vi "Actor Core.vi"(8 "error in":errorcluster, 11 "Gui in":refnum<class "Gui.lvclass">) -> (0 "error out":errorcluster, 3 "Actor out":refnum<class "Actor.lvclass">)   [LabVIEW 2022 SP3, in "Gui.lvlib" / "Gui.lvclass"]
doc: "(<B>Filename</B>: Actor Framework.lvlib:Actor.lvclass:Actor Core.vi)\n\nReceives messages to the actor, reacts to them, and initiates any error handling that may shut the actor down.\n\nDescendant classes may override this VI to append parallel tasks for the actor to complete while it handles messages. Overrides use the Call Parent Class Method node."
uses:
  Gui.lvclass
  C:/Program Files (x86)/National Instruments/LabVIEW 2022/vi.lib/ActorFramework/Actor/Actor.lvclass
  <vilib>/ActorFramework/Actor/Actor.lvclass
  Gui.lvclass/Gui.ctl
  <vilib>/ActorFramework/Actor/Actor.lvclass/Actor.ctl
  <vilib>/ActorFramework/Message Enqueuer/Message Enqueuer.lvclass/Message Enqueuer.ctl
  <vilib>/ActorFramework/Message Enqueuer/Init from Existing Queue.vi
  <vilib>/ActorFramework/Message Enqueuer/Enqueue.vi
  CallerMessage Messages/GuiPanelClose Msg/GuiPanelClose Msg.lvclass
  C:/Program Files (x86)/National Instruments/LabVIEW 2022/vi.lib/ActorFramework/Message/Message.lvclass
  <vilib>/ActorFramework/Message Priority Queue/Priority Enqueue.vi
  <vilib>/ActorFramework/Message Enqueuer/Message Enqueuer.lvclass
panel:
  out "Uptime [s]":string
  # "<< GUI >>"
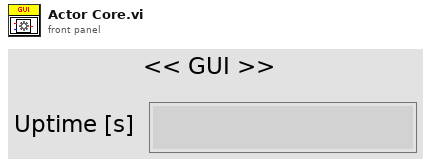
[diagram p1: front panel]
types:
  T1 = typedef "Gui.lvlib/Gui.lvclass/_Events.ctl" = cluster{"StopGuiLoop":refnum<user-event>}
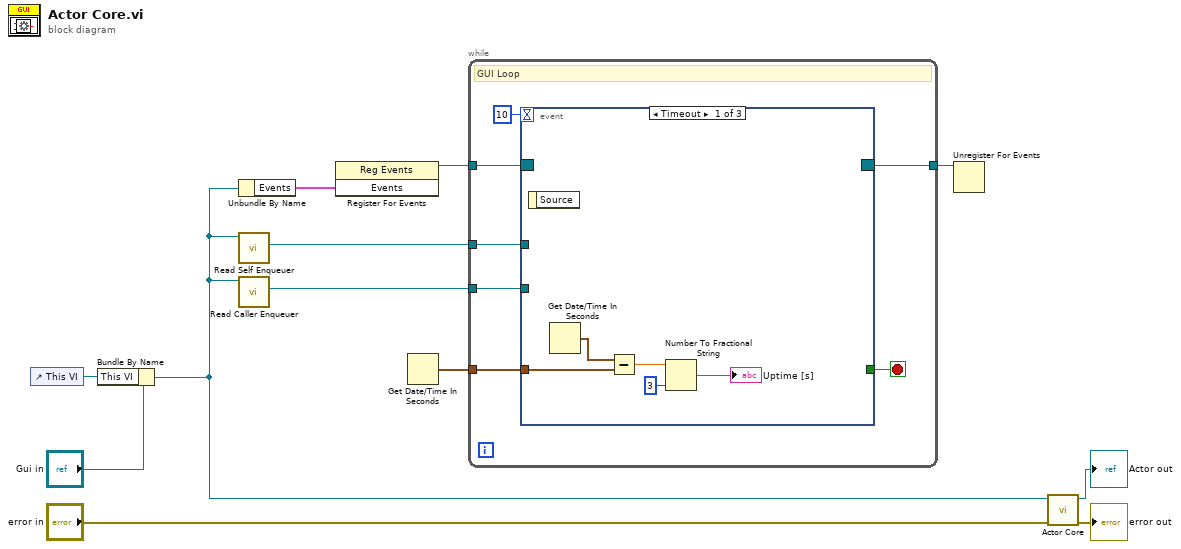
[diagram p0: block diagram]
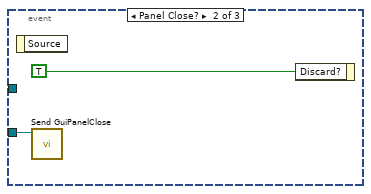
[diagram p2: hidden frame]
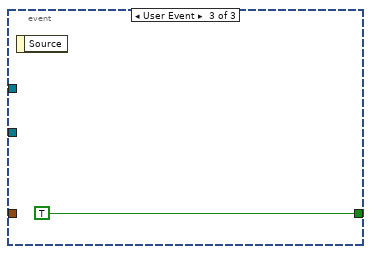
[diagram p3: hidden frame]
diagram:
  n1 = control-ref of="This VI"() -> (w4:refnum<vi>)
  n2 = Bundle By Name(cluster="Gui in", "This VI"=w4) -> (w2:refnum<class "Gui.lvclass">)
  n3 = Unbundle By Name(w2) -> ("Events"=w7:T1)
  n4 = call <vilib>:"Read Self Enqueuer.vi"("Actor"=w2) -> ("Self Enqueuer"=w8:refnum<class "Message Enqueuer.lvclass">)  [unwired: 10 in]
  n5 = call <vilib>:"Read Caller Enqueuer.vi"("Actor"=w2) -> ("Caller Enqueuer"=w9:refnum<class "Message Enqueuer.lvclass">)  [unwired: 10 in]
  n6 = register-events(w7) -> (reference out=w6:refnum<event-registration>)  [unwired: 2 in, 1 out]
  n7 = Get Date/Time In Seconds() -> (seconds since 1Jan1904=w1:timestamp)
  n8 = while {
    tunnel: w9 -> [w19]
    tunnel: w8 -> [w18]
    tunnel: w6 -> [w17]
    tunnel: [w16] -> w5
    tunnel: w1 -> [w13]
    stop <- w15 stop-if-true
    # "GUI Loop"
    n9 = event shown="[0] Timeout" {
      selector: w17 -> [_ _ _]
      dyn-events: [_ _ _] -> w16
      timeout: 10 -> [_ _ _]
      tunnel: w19 -> [_ w25 _]
      tunnel: w18 -> [_ _ _]
      tunnel: [_ _ TRUE] -> w15
      tunnel: w13 -> [w23 _ _]
      event Timeout {
        n10 = event-data() -> ()  [unwired: 1 in, 1 out]
        n11 = Get Date/Time In Seconds() -> (seconds since 1Jan1904=w24:timestamp)
        n12 = Subtract(x=w24, y=w23) -> (x-y=w22:dbl)
        n13 = Number To Fractional String(number=w22, precision (6)=i16 3) -> (F-format string=→"Uptime [s]":string)  [unwired: 2 in]
      }
      event Panel Close? {
        n14 = event-data() -> ()  [unwired: 1 in, 1 out]
        n15 = call "Send GuiPanelClose.vi"("Message Enqueuer"=w25) -> ()  [unwired: 9 in, 2 out]
        n16 = event-data("Discard?"=TRUE) -> ()  [unwired: 1 in, 1 out]
      }
      event User Event {
        n17 = event-data() -> ()  [unwired: 1 in, 1 out]
      }
    }
  }
  n18 = Unregister For Events(event registration refnum=w5) -> ()  [unwired: 1 in, 1 out]
  n19 = call-parent "Actor Core.vi"("error in"="error in", "Actor in"=w2) -> ("error out"=→"error out":errorcluster, "Actor out"=→"Actor out":refnum<class "Actor.lvclass">)  [unwired: 8 in]
